vi "Subscribe.vi"(8 "error in (no error)":errorcluster, 9 "Subscriber Enqueuer":refnum<class "Message Enqueuer.lvclass">, 10 "Topic":string, 11 "Broadcaster in":refnum<class "BroadcastBroker.lvclass">) -> (0 "error out":errorcluster, 3 "Broadcaster out":refnum<class "BroadcastBroker.lvclass">)   [LabVIEW 2015, in "BroadcastBroker.lvclass"]
uses:
  BroadcastBroker.lvclass
  <vilib>/ActorFramework/Message Enqueuer/Message Enqueuer.lvclass
  BroadcastBroker.lvclass/BroadcastBroker.ctl
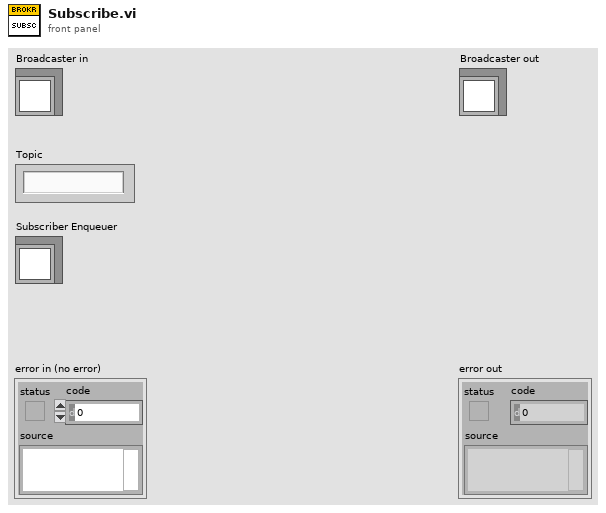
[diagram p1: front panel]
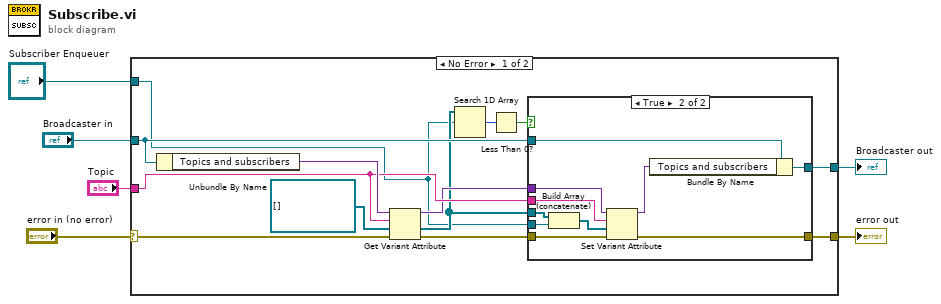
[diagram p0: block diagram]
diagram:
  n1 = case shown="No Error" "error in (no error)" {
    selector: "error in (no error)" -> [w17 w33]
    tunnel: [w11 w33] -> w5
    tunnel: [w12 w32] -> w3
    tunnel: "Broadcaster in" -> [w19 w32]
    tunnel: "Topic" -> [w15 _]
    tunnel: "Subscriber Enqueuer" -> [w9 _]
    frame No Error {
      n2 = Unbundle By Name(w19) -> ("Topics and subscribers"=w18:variant)
      n3 = Get Variant Attribute(Variant=w18, name=w15, default value (empty Variant)=refnum<class "Message Enqueuer.lvclass">[] [], error in=w17) -> (duplicate Variant=w13:variant, value=w10:refnum<class "Message Enqueuer.lvclass">[], error out=w14:errorcluster)  [unwired: 1 out]
      n4 = Search 1D Array(1D array=w10, element=w9) -> (index of element=w8:i32)  [unwired: 1 in]
      n5 = Less Than 0?(x=w8) -> (x < 0?=w7:bool)
      n6 = case shown="True" w7 {
        tunnel: w19 -> [w21 w31]
        tunnel: w15 -> [_ w30]
        tunnel: w14 -> [w20 w29]
        tunnel: w13 -> [_ w27]
        tunnel: [w21 w26] -> w12
        tunnel: [w20 w24] -> w11
        tunnel: w10 -> [_ w23]
        tunnel: w9 -> [_ w22]
        frame False {
        }
        frame True {
          n7 = Build Array (concatenate)(w23, w22) -> (w28:refnum<class "Message Enqueuer.lvclass">[])
          n8 = Set Variant Attribute(Variant=w27, name=w30, value=w28, error in=w29) -> (Variant out=w25:variant, error out=w24:errorcluster)  [unwired: 1 out]
          n9 = Bundle By Name(cluster=w31, "Topics and subscribers"=w25) -> (w26:refnum<class "BroadcastBroker.lvclass">)
        }
      }
    }
    frame Error {
    }
  }
  "error out" <- w5
  "Broadcaster out" <- w3
